vi "Create Folder If Misssing.vi"(2 "error in":errorcluster, 3 "Path In":path) -> (0 "error out":errorcluster, 1 "Path Out":path)   [LabVIEW 2018]
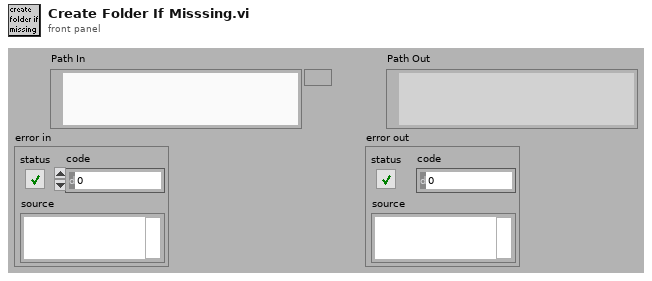
[diagram p1: front panel]
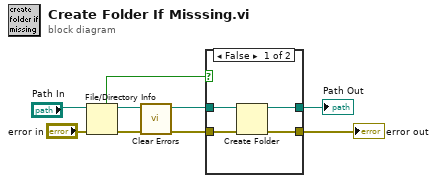
[diagram p0: block diagram]
diagram:
  n1 = File/Directory Info(path="Path In", error in="error in") -> (path out=w6:path, directory=w7:bool, error out=w2:errorcluster)  [unwired: 4 out]
  n2 = call <vilib>:"Clear Errors.vi"("error in (no error)"=w2) -> ("error out"=w1:errorcluster)  [unwired: 5 in, 1 out]
  n3 = case shown="False" w7 {
    tunnel: w6 -> [w12 w14]
    tunnel: [w11 w14] -> w5
    tunnel: w1 -> [w10 w13]
    tunnel: [w9 w13] -> w4
    frame False {
      n4 = Create Folder(path (use dialog)=w12, error in=w10) -> (created path=w11:path, error out=w9:errorcluster)  [unwired: 1 in, 1 out]
    }
    frame True {
      # "directory\ndoes not exist"
    }
  }
  "Path Out" <- w5
  "error out" <- w4
